vi "Test Message Manager 1.vi"(11 "Test Case In":refnum<class "PCAN Tests.lvclass">) -> (0 "error out":errorcluster, 3 "Test Case Out":refnum<class "PCAN Tests.lvclass">)   [LabVIEW 2025, in "PCAN Tests.lvclass"]
uses:
  PCAN Tests.lvclass
  PCAN Tests.lvclass/PCAN Tests.ctl
  4993e8ee-a06a-463a-9684-69129f64d5ce.vi
  Messaging Buffer/Message Buffer.lvclass
  Interfaces/IMessage/IMessage.lvclass
panel:
  out "Messages":refnum<class "IMessage.lvclass">[][](array[class])
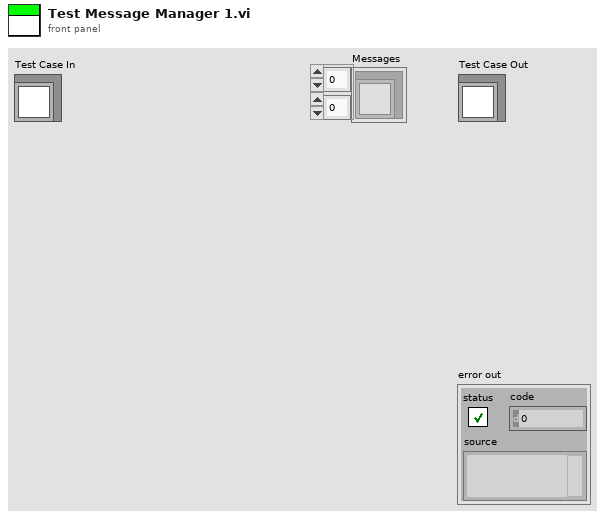
[diagram p1: front panel]
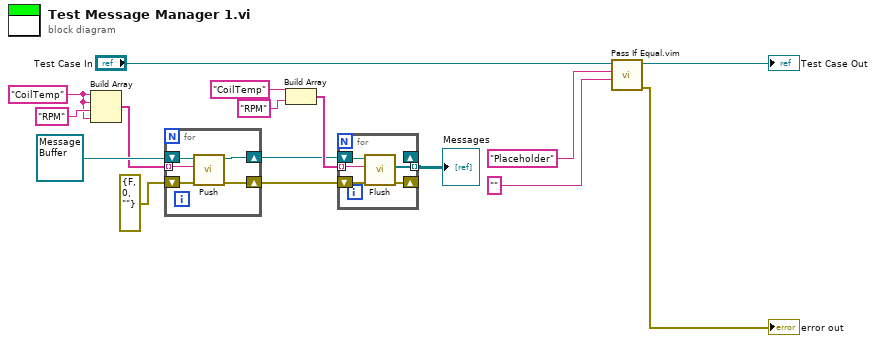
[diagram p0: block diagram]
diagram:
  w8 = "CoilTemp" ("Receiver ID")
  n1 = Build Array(w8, w8, "RPM" ("Receiver ID"), w8) -> (w10:string[])
  n2 = for {
    tunnel: w10 -> [w20] mode=indexing
    shift-right: [w18] -> w6
    shift-left: errorcluster {"status"=FALSE, "code"=0, "source"=""} ("error constant") -> [w19]
    shift-right: [w17] -> w2
    shift-left: refnum<class "Message Buffer.lvclass"> refnum ("PCAN.lvlib:Messaging Manager.lvclass") -> [w21]
    n3 = call "Push.vi"("error in"=w19, "IMessage"=w20, "Message Buffer in"=w21) -> ("error out"=w18:errorcluster, "Message Buffer out"=w17:refnum<class "Message Buffer.lvclass">)  [unwired: 7 in]
  }
  n4 = Build Array("CoilTemp" ("Receiver ID"), "RPM" ("Receiver ID")) -> (w3:string[])
  n5 = for {
    tunnel: w3 -> [w25] mode=indexing
    shift-right: _ -> [_]
    shift-left: w2 -> [w24]
    shift-right: [w23] -> _
    shift-left: w6 -> [w26]
    tunnel: [w22] -> w1 mode=indexing
    n6 = call "Flush.vi"("error in"=w26, 10:w25, "Message Buffer in"=w24) -> ("error out"=w23:errorcluster, "Messages"=w22:refnum<class "IMessage.lvclass">[])  [unwired: 6 in, 1 out]
  }
  "Messages" <- w1
  n7 = call "Pass If Equal.vim"("Actual"="", "Expected"="Placeholder", "LUnit Test Case In"="Test Case In") -> ("error out"=→"error out":errorcluster, "LUnit Test Case Out"=→"Test Case Out":refnum<class "PCAN Tests.lvclass">)  [unwired: 7 in]
